vi "Z to dB, degrees (2D).vi"(6 "Z":cdb[][](array[numeric])) -> (1 "Magnitude (dB)":dbl[][](array[numeric]), 2 "Phase (degrees)":dbl[][](array[numeric]))   [LabVIEW 2020]
uses:
  ab3eb4fe-677d-43fd-b108-0463c1fb254e.vi
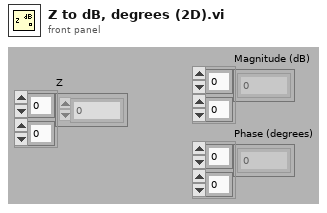
[diagram p1: front panel]
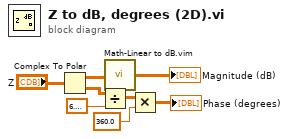
[diagram p0: block diagram]
diagram:
  n1 = Complex To Polar(r * e^(i*theta)="Z") -> (r=w7:dbl[][], theta=w6:dbl[][])
  n2 = Divide(x=w6, y=6.283185307179586) -> (x/y=w4:dbl[][])
  n3 = call "Math-Linear to dB.vim"("linear"=w7) -> ("dB"=→"Magnitude (dB)":dbl[][])
  n4 = Multiply(x=w4, y=360.0) -> (x*y=→"Phase (degrees)":dbl[][])
